vi "全局 3.vi"() -> ()   [LabVIEW 2012]
panel:
  in  "总合格状态":string
  in  "合格判断":string
  in  "stop":bool
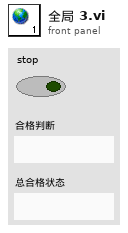
[diagram p1: front panel]
diagram:
